vi "Update Config File Section (Subsystem).vi"(7 "UpdatedConfigSection (Subsystem)":variant, 8 "error in (no error)":errorcluster, 9 "Configuration (Full Cluster)":variant, 10 "XML File Path":path, 11 "Config in":refnum<class "Config.lvclass">) -> (0 "error out":errorcluster, 1 "Configuration out":variant, 2 "XML File Path out":path, 3 "Config out":refnum<class "Config.lvclass">, 4 "Section Not found?":bool, 5 "Section (Subsystem) Data Name":string)   [LabVIEW 2019, in "Config.lvclass"]
doc: "Developed by Kevin Thompson\nkevin@thompsonengineering.net\n\nCopyright 2020\nThompson Engineering, LLC"
uses:
  Config.lvclass
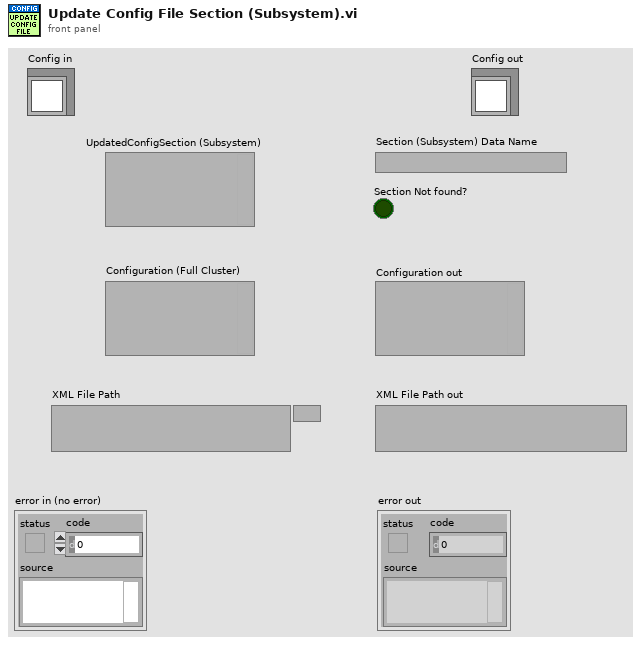
[diagram p1: front panel]
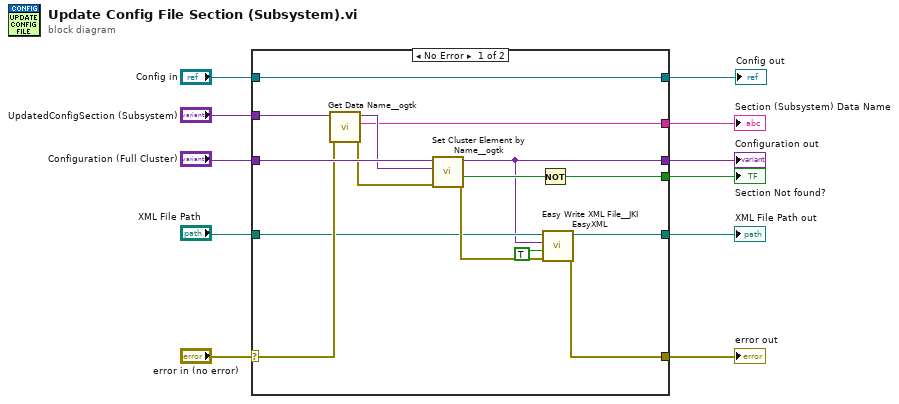
[diagram p0: block diagram]
diagram:
  n1 = case shown="No Error" "error in (no error)" {
    selector: "error in (no error)" -> [w20 w30]
    tunnel: [w19 w30] -> w10
    tunnel: "Configuration (Full Cluster)" -> [w25 w29]
    tunnel: "UpdatedConfigSection (Subsystem)" -> [w26 _]
    tunnel: "XML File Path" -> [w18 w28]
    tunnel: [w17 w28] -> w6
    tunnel: [w15 _] -> w5
    tunnel: [w14 _] -> w4
    tunnel: [w13 w29] -> w3
    tunnel: [w12 w27] -> w1
    tunnel: "Config in" -> [w12 w27]
    frame No Error {
      n2 = call <userlib>:"Get Data Name__ogtk.vi"("error in (no error)"=w20, "Data"=w26) -> ("error out"=w23:errorcluster, "Data Name"=w14:string, "Data dup"=w24:variant)  [unwired: 7 in]
      n3 = call <userlib>:"Set Cluster Element by Name__ogtk.vi"("error in (no error)"=w23, "New Element Value"=w24, "Cluster"=w25) -> ("error out"=w21:errorcluster, "found?"=w16:bool, "VCluster out"=w13:variant)  [unwired: 6 in]
      n4 = Not(x=w16) -> (.not. x?=w15:bool)
      n5 = call <vilib>:"Easy Write XML File__JKI EasyXML.vi"("error in (no error)"=w21, "Overwrite File? (false)"=TRUE, "LabVIEW Data"=w13, "XML File Path"=w18) -> ("error out"=w19:errorcluster, "XML File Path (duplicate)"=w17:path)  [unwired: 6 in]
    }
    frame Error {
    }
  }
  "error out" <- w10
  "XML File Path out" <- w6
  "Section Not found?" <- w5
  "Section (Subsystem) Data Name" <- w4
  "Configuration out" <- w3
  "Config out" <- w1
